vi "LSX Get Snapshot Par.vi"(8 "error in (no error)":errorcluster, 9 "pbAutoMode":i32, 10 "pbHigh":i32, 11 "lLSID":i32) -> (0 "error out":errorcluster, 1 "pbAutoMode out":i32, 2 "pbHigh out":i32, 3 "function return":i32)   [LabVIEW 2018, in "Tango.lvlib"]
doc: "TANGOAPI int TANGOCALL LSX_GetSnapshotPar (int lLSID, BOOL *pbHigh, BOOL *pbAutoMode);"
uses:
  Tango.lvlib
  SubVIs/Tango_DLL.dll
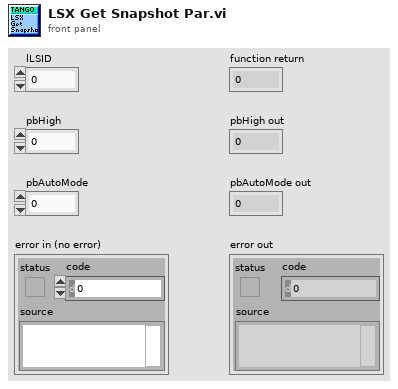
[diagram p1: front panel]
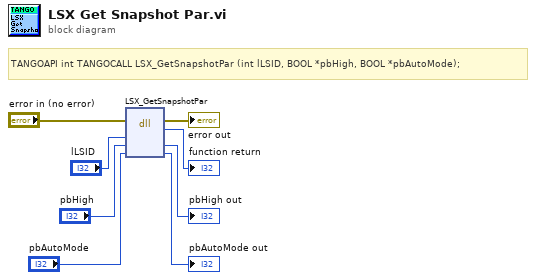
[diagram p0: block diagram]
diagram:
  # "TANGOAPI int TANGOCALL LSX_GetSnapshotPar (int lLSID, BOOL *pbHigh, BOOL *pbAutoMode);"
  n1 = dll-call lib="C:/Users/Familie/Documents/LabviewIX81/lib/TANGO Stage/SubVIs/Tango_DLL.*" fn="LSX_GetSnapshotPar"(error in="error in (no error)", "lLSID"="lLSID", "pbHigh"="pbHigh", "pbAutoMode"="pbAutoMode") -> (error out=→"error out":errorcluster, →"function return":i32, "pbHigh"=→"pbHigh out":i32, "pbAutoMode"=→"pbAutoMode out":i32)  [unwired: 3 in, 1 out]
